vi "Pilih Kalibrasi - v04.vi"(0 "Kalibrasi":T2(ring), 5 "Default":bool, 7 "Min In":dbl, 9 "Max In":dbl, 11 "Input":dbl) -> (3 "Ind.Col":i32, 4 "Max Input":dbl, 6 "Min Input":dbl, 8 "Min Data Kalibrasi":dbl, 10 "Max Data Kalibrasi":dbl, 13 "Disabled Items []":i32[](array[numeric]), 14 "MaxMinEnabled":T1(ring), 15 "Data Kalibrasi":dbl)   [LabVIEW 2018]
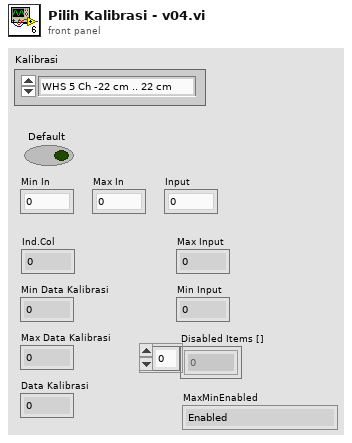
[diagram p1: front panel]
types:
  T1 = enum8{"Enabled", "Disabled", "Disabled and Grayed Out"}
  T2 = enum16{"WHS 5 Ch -22 cm .. 22 cm", "WHS 5 Ch -20 cm .. 20 cm", "WHS 1 Ch -20 cm .. 20 cm", "R-56 Resistance", "H-39 Open Water Thrust", "H-39 Open Water Torsi CW", "H-39 Open Water Torsi CCW", "R-31 Self Propulsi Thrust", "R-31 Self Propulsi Torsi CW", "R-31 Self Propulsi Torsi CCW", "R-33 Self Propulsi Thrust", "R-33 Self Propulsi Torsi CW", "R-33 Self Propulsi CCW", "Other Sensor Data"}
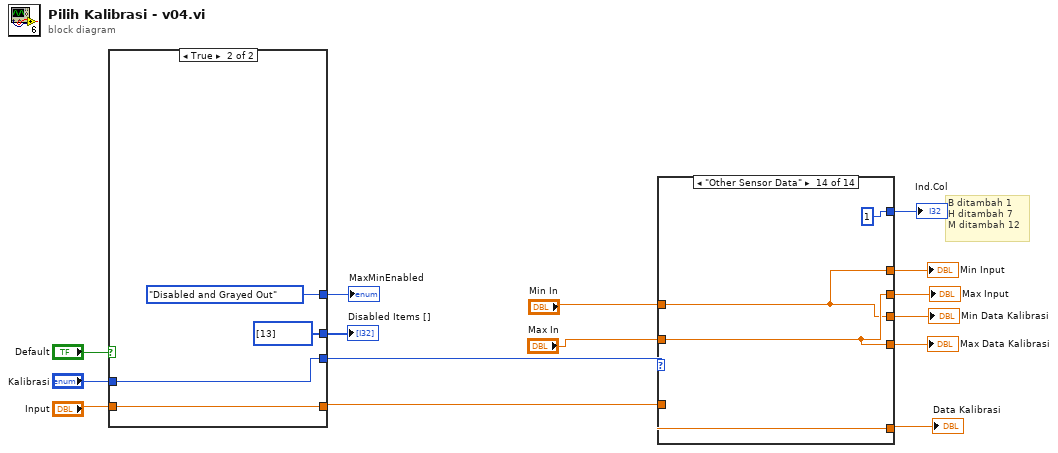
[diagram p0: block diagram]
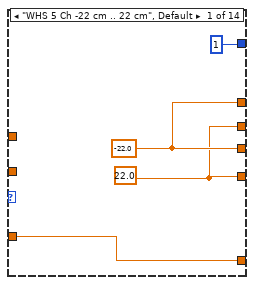
[diagram p2: hidden frame]
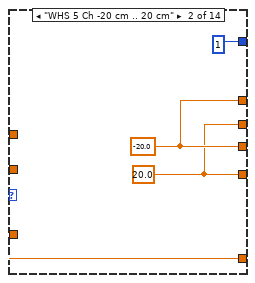
[diagram p3: hidden frame]
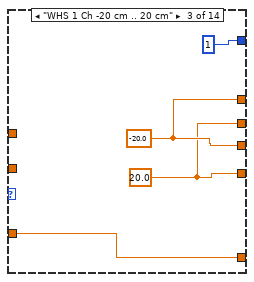
[diagram p4: hidden frame]
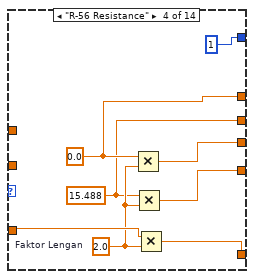
[diagram p5: hidden frame]
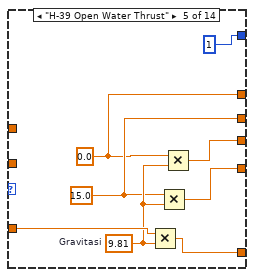
[diagram p6: hidden frame]
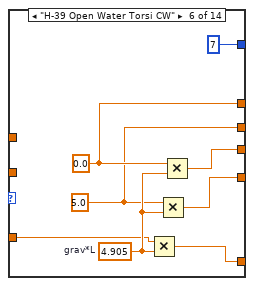
[diagram p7: hidden frame]
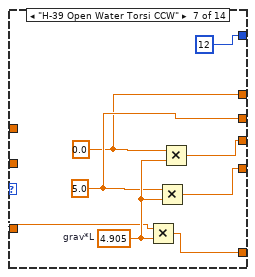
[diagram p8: hidden frame]
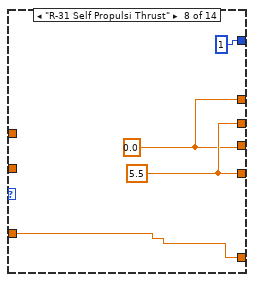
[diagram p9: hidden frame]
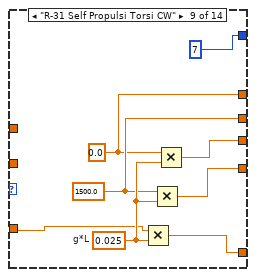
[diagram p10: hidden frame]
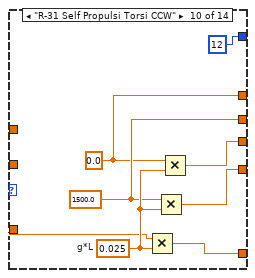
[diagram p11: hidden frame]
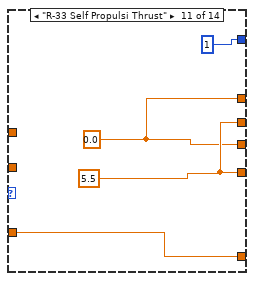
[diagram p12: hidden frame]
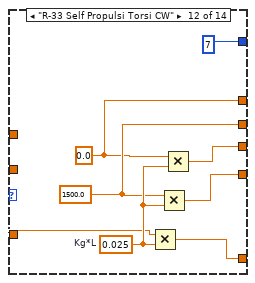
[diagram p13: hidden frame]
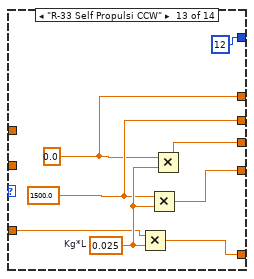
[diagram p14: hidden frame]
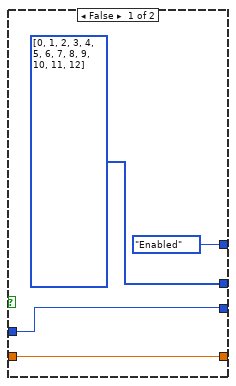
[diagram p15: hidden frame]
diagram:
  # "B ditambah 1\nH ditambah 7\nM ditambah 12"
  n1 = case shown="True" "Default" {
    tunnel: [w17 w21] -> w14
    tunnel: "Kalibrasi" -> [w17 w21]
    tunnel: [w19 w23] -> w13
    tunnel: "Input" -> [w19 w23]
    tunnel: [T1."Enabled" ("Disabled") T1."Disabled and Grayed Out" ("Disabled")] -> w8
    tunnel: [i32[] [0, 1, 2, 3, 4, 5, 6, 7, 8, 9, 10, 11, 12] ("Disabled Items []") i32[] [13] ("Disabled Items []")] -> w6
    frame False {
    }
    frame True {
    }
  }
  "Disabled Items []" <- w6
  "MaxMinEnabled" <- w8
  n2 = case shown="\"Other Sensor Data\"" w14 {
    tunnel: [w26 w30 w34 w39 w47 w57 w62 w69 w77 w86 w89 w98 w106 w109] -> w9
    tunnel: [w25 w29 w33 w40 w49 w56 w61 w70 w76 w85 w90 w97 w105 w110] -> w10
    tunnel: w13 -> [w27 w31 w35 w42 w51 w58 w66 w71 w78 w83 w91 w95 w103 w111]
    tunnel: [w27 w31 w35 w43 w50 w55 w65 w71 w75 w84 w91 w96 w104 w111] -> w11
    tunnel: "Min In" -> [_ _ _ _ _ _ _ _ _ _ _ _ _ w109]
    tunnel: "Max In" -> [_ _ _ _ _ _ _ _ _ _ _ _ _ w110]
    tunnel: [1 1 1 1 1 7 12 1 7 12 1 7 12 1] -> w7
    tunnel: [w26 w30 w34 w38 w45 w54 w63 w69 w73 w81 w89 w93 w101 w109] -> w3
    tunnel: [w25 w29 w33 w37 w46 w53 w64 w70 w74 w82 w90 w94 w102 w110] -> w2
    frame "WHS 5 Ch -22 cm .. 22 cm", Default {
      w25 = 22.0 ("Min")
      w26 = -22.0 ("Min")
    }
    frame "WHS 5 Ch -20 cm .. 20 cm" {
      w29 = 20.0 ("Min")
      w30 = -20.0 ("Min")
    }
    frame "WHS 1 Ch -20 cm .. 20 cm" {
      w33 = 20.0 ("Min")
      w34 = -20.0 ("Min")
    }
    frame "R-56 Resistance" {
      w41 = 2.0  # Faktor Lengan
      w37 = 15.488 ("Min")
      w38 = 0.0 ("Min")
      n3 = Multiply(x=w38, y=w41) -> (x*y=w39:dbl)
      n4 = Multiply(x=w37, y=w41) -> (x*y=w40:dbl)
      n5 = Multiply(x=w42, y=w41) -> (x*y=w43:dbl)
    }
    frame "H-39 Open Water Thrust" {
      w48 = 9.81  # Gravitasi
      w46 = 15.0 ("Min")
      w45 = 0.0 ("Min")
      n6 = Multiply(x=w51, y=w48) -> (x*y=w50:dbl)
      n7 = Multiply(x=w46, y=w48) -> (x*y=w49:dbl)
      n8 = Multiply(x=w45, y=w48) -> (x*y=w47:dbl)
    }
    frame "H-39 Open Water Torsi CW" {
      w59 = 4.905  # grav*L
      w53 = 5.0 ("Min")
      w54 = 0.0 ("Min")
      n9 = Multiply(x=w58, y=w59) -> (x*y=w55:dbl)
      n10 = Multiply(x=w53, y=w59) -> (x*y=w56:dbl)
      n11 = Multiply(x=w54, y=w59) -> (x*y=w57:dbl)
    }
    frame "H-39 Open Water Torsi CCW" {
      w67 = 4.905  # grav*L
      w64 = 5.0 ("Min")
      w63 = 0.0 ("Min")
      n12 = Multiply(x=w66, y=w67) -> (x*y=w65:dbl)
      n13 = Multiply(x=w64, y=w67) -> (x*y=w61:dbl)
      n14 = Multiply(x=w63, y=w67) -> (x*y=w62:dbl)
    }
    frame "R-31 Self Propulsi Thrust" {
      w70 = 5.5 ("Min")
      w69 = 0.0 ("Min")
    }
    frame "R-31 Self Propulsi Torsi CW" {
      w79 = 0.025  # g*L
      w74 = 1500.0 ("Min")
      w73 = 0.0 ("Min")
      n15 = Multiply(x=w78, y=w79) -> (x*y=w75:dbl)
      n16 = Multiply(x=w74, y=w79) -> (x*y=w76:dbl)
      n17 = Multiply(x=w73, y=w79) -> (x*y=w77:dbl)
    }
    frame "R-31 Self Propulsi Torsi CCW" {
      w87 = 0.025  # g*L
      w82 = 1500.0 ("Min")
      w81 = 0.0 ("Min")
      n18 = Multiply(x=w83, y=w87) -> (x*y=w84:dbl)
      n19 = Multiply(x=w82, y=w87) -> (x*y=w85:dbl)
      n20 = Multiply(x=w81, y=w87) -> (x*y=w86:dbl)
    }
    frame "R-33 Self Propulsi Thrust" {
      w90 = 5.5 ("Min")
      w89 = 0.0 ("Min")
    }
    frame "R-33 Self Propulsi Torsi CW" {
      w99 = 0.025  # Kg*L
      w94 = 1500.0 ("Min")
      w93 = 0.0 ("Min")
      n21 = Multiply(x=w95, y=w99) -> (x*y=w96:dbl)
      n22 = Multiply(x=w94, y=w99) -> (x*y=w97:dbl)
      n23 = Multiply(x=w93, y=w99) -> (x*y=w98:dbl)
    }
    frame "R-33 Self Propulsi CCW" {
      w107 = 0.025  # Kg*L
      w102 = 1500.0 ("Min")
      w101 = 0.0 ("Min")
      n24 = Multiply(x=w103, y=w107) -> (x*y=w104:dbl)
      n25 = Multiply(x=w102, y=w107) -> (x*y=w105:dbl)
      n26 = Multiply(x=w101, y=w107) -> (x*y=w106:dbl)
    }
    frame "Other Sensor Data" {
    }
  }
  "Max Data Kalibrasi" <- w10
  "Min Data Kalibrasi" <- w9
  "Data Kalibrasi" <- w11
  "Min Input" <- w3
  "Max Input" <- w2
  "Ind.Col" <- w7
